vi "WLAN_SigBuild - 2SC.vi"(0 "Data bit length":i32, 1 "Modulation parameter":T1, 3 "error in (no error)":errorcluster) -> (7 "symbols":cdb[](array[numeric]) format="%.3f", 10 "error out":errorcluster)   [LabVIEW 2022 SP3]
panel:
  out "output array":i8[](array[numeric])
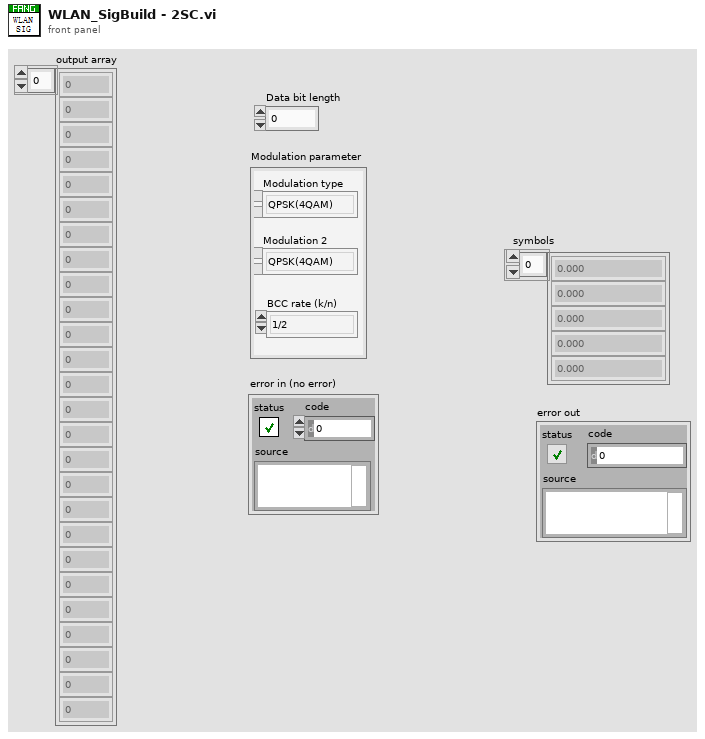
[diagram p1: front panel]
types:
  T1 = cluster{"Modulation type":enum16{"QPSK(4QAM)", "64QAM", "16QAM", "BPSK", "BPSK Vertical"}, "BCC rate (k/n)":enum16{"1/2", "2/3", "3/4"}, "Modulation 2":enum16{"QPSK(4QAM)", "64QAM", "16QAM", "BPSK", "BPSK Vertical"}}
  T2 = enum16{"QPSK(4QAM)", "64QAM", "16QAM", "BPSK", "BPSK Vertical"}
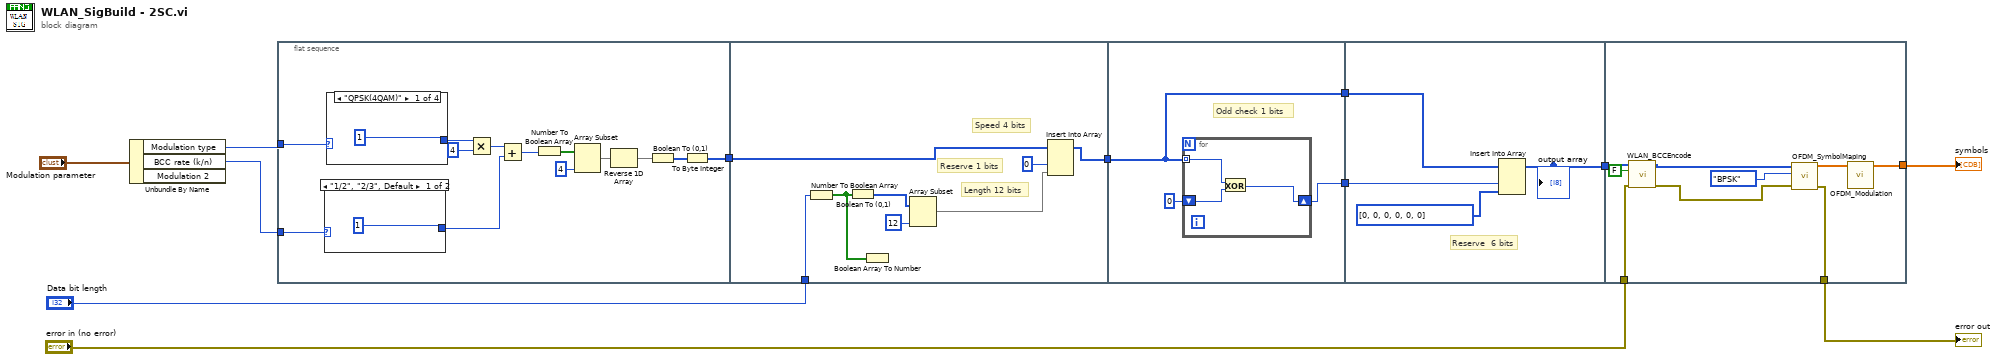
[diagram p0: block diagram]
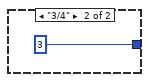
[diagram p2: hidden frame]
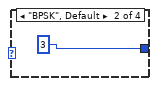
[diagram p3: hidden frame]
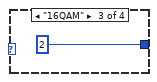
[diagram p4: hidden frame]
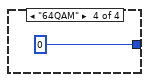
[diagram p5: hidden frame]
diagram:
  n1 = Unbundle By Name("Modulation parameter") -> ("Modulation type"=w12:T2, "BCC rate (k/n)"=w11:enum16{"1/2", "2/3", "3/4"})  [unwired: 1 out]
  n2 = flat-sequence {
    tunnel: w12 -> [w15]
    tunnel: w11 -> [w14]
    tunnel: [w13] -> w10
    tunnel: w10 -> [w34]
    tunnel: "Data bit length" -> [w33]
    tunnel: [w32] -> w8
    tunnel: w8 -> [w41]
    tunnel: [w42] -> w7
    tunnel: [w41] -> w6
    tunnel: w7 -> [w48]
    tunnel: w6 -> [w47]
    tunnel: [w46] -> w5
    tunnel: w5 -> [w55]
    tunnel: "error in (no error)" -> [w54]
    tunnel: [w52] -> w3
    tunnel: [w51] -> w2
    frame #0 {
      n3 = case shown="\"1/2\", \"2/3\", Default" w14 {
        tunnel: [1 3] -> w19
        frame "1/2", "2/3", Default {
        }
        frame "3/4" {
        }
      }
      n4 = case shown="\"QPSK(4QAM)\"" w15 {
        tunnel: [1 3 2 0] -> w16
        frame "QPSK(4QAM)" {
        }
        frame "BPSK", Default {
        }
        frame "16QAM" {
        }
        frame "64QAM" {
        }
      }
      n5 = Multiply(x=w16, y=4) -> (x*y=w18:i32)
      n6 = Add(x=w18, y=w19) -> (x+y=w20:i32)
      n7 = Number To Boolean Array(number=w20) -> (Boolean array=w21:bool[])
      n8 = Array Subset(array=w21, length=4) -> (w23:bool[])  [unwired: 1 in]
      n9 = Reverse 1D Array(array=w23) -> (reversed array=w24:bool[])
      n10 = Boolean To (0,1)(Boolean=w24) -> (0, 1=w25:i16[])
      n11 = To Byte Integer(number=w25) -> (8bit integer=w13:i8[])
    }
    frame #1 {
      # "Length 12 bits"
      # "Reserve 1 bits"
      # "Speed 4 bits"
      n12 = Number To Boolean Array(number=w33) -> (Boolean array=w39:bool[])
      n13 = Boolean To (0,1)(Boolean=w39) -> (0, 1=w36:i16[])
      n14 = Boolean Array To Number(Boolean array=w39) -> ()  [unwired: 1 out]
      n15 = Array Subset(array=w36, length=12) -> (w38:i16[])  [unwired: 1 in]
      n16 = Insert Into Array(array=w34, new element #1=i8 0 ("new element/subarray"), new element #2=w38) -> (w32:i8[])  [unwired: 1 in]
    }
    frame #2 {
      # "Odd check 1 bits"
      n17 = for {
        tunnel: w41 -> [w45] mode=indexing
        shift-right: [w43] -> w42
        shift-left: i8 0 -> [w44]
        n18 = Exclusive Or(1:w44, 2:w45) -> (0:w43:i8)
      }
    }
    frame #3 {
      # "Reserve  6 bits"
      n19 = Insert Into Array(array=w47, new element #1=w48, new element #2=i8[] [0, 0, 0, 0, 0, 0]) -> (w46:i8[])  [unwired: 1 in]
      "output array" <- w46
    }
    frame #4 {
      n20 = call "WLAN_BCCEncode.vi"("error in (no error)"=w54, "need add zeros?"=FALSE, "input bit stream"=w55) -> ("error out"=w57:errorcluster, "output bit stream 3"=w58:i8[])  [unwired: 7 in]
      n21 = call "OFDM_SymbolMaping.vi"("error in (no error)"=w57, "Modulation type"=enum16{"QPSK(4QAM)", "64QAM", "16QAM", "BPSK"}."BPSK", "input bit stream"=w58) -> ("error out"=w52:errorcluster, "symbols"=w53:cdb[])  [unwired: 7 in]
      n22 = call "OFDM_Modulation.vi"("Input sequence"=w53) -> ("Output sequence"=w51:cdb[])  [unwired: 10 in]
    }
  }
  "symbols" <- w2
  "error out" <- w3
